vi "Write Status Updated Msg.vi"(10 "Chat Window Model.lvlib:Status Updated Msg.lvclass":refnum<class "Status Updated Msg.lvclass">, 11 "Chat Window Model in":refnum<class "Chat Window Model.lvclass">) -> (3 "Chat Window Model out":refnum<class "Chat Window Model.lvclass">)   [LabVIEW 2015, in "Chat Window Model.lvlib" / "Chat Window Model.lvclass"]
uses:
  Chat Window Model.lvclass
  Chat Window Model Messages/Status Updated Msg/Status Updated Msg.lvclass
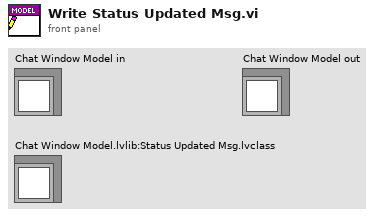
[diagram p1: front panel]
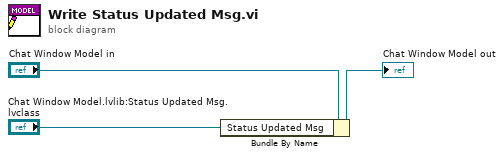
[diagram p0: block diagram]
diagram:
  n1 = Bundle By Name(cluster="Chat Window Model in", "Status Updated Msg"="Chat Window Model.lvlib:Status Updated Msg.lvclass") -> (→"Chat Window Model out":refnum<class "Chat Window Model.lvclass">)
